vi "Make DLL Param(Read Batch Profile Rsp).vi"(1 "Read Batch Profile Rsp":T1) -> (0 "pRsp":T2)   [LabVIEW 2015, in "KEYENCE LJ-X8000A.lvlib"]
uses:
  KEYENCE LJ-X8000A.lvlib
  Public/Clusters/Read Batch Profile Rsp.ctl
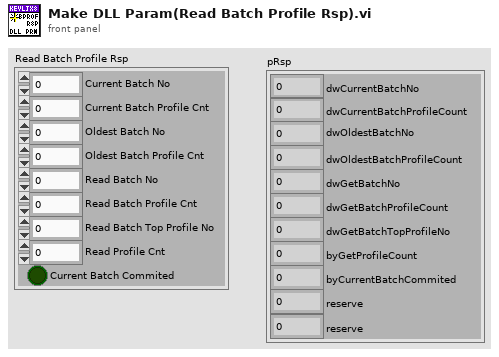
[diagram p1: front panel]
types:
  T1 = typedef "KEYENCE LJ-X8000A.lvlib/Read Batch Profile Rsp.ctl" = cluster{"Current Batch No":u32, "Current Batch Profile Cnt":u32, "Oldest Batch No":u32, "Oldest Batch Profile Cnt":u32, "Read Batch No":u32, "Read Batch Profile Cnt":u32, "Read Batch Top Profile No":u32, "Read Profile Cnt":u32, "Current Batch Commited":bool}
  T2 = cluster{"dwCurrentBatchNo":u32, "dwCurrentBatchProfileCount":u32, "dwOldestBatchNo":u32, "dwOldestBatchProfileCount":u32, "dwGetBatchNo":u32, "dwGetBatchProfileCount":u32, "dwGetBatchTopProfileNo":u32, "byGetProfileCount":u8, "byCurrentBatchCommited":u8, "reserve":u8, "reserve":u8}
  T3 = cluster{"Current Batch No":u32, "Current Batch Profile Cnt":u32, "Oldest Batch No":u32, "Oldest Batch Profile Cnt":u32, "Read Batch No":u32, "Read Batch Profile Cnt":u32, "Read Batch Top Profile No":u32, "Read Profile Cnt":u32, u8, "reserve":u8, "reserve":u8}
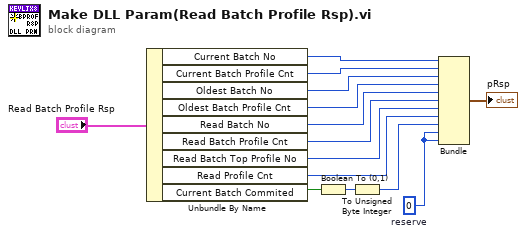
[diagram p0: block diagram]
diagram:
  w5 = u8 0  # reserve
  n1 = Unbundle By Name("Read Batch Profile Rsp") -> ("Current Batch No"=w14:u32, "Current Batch Profile Cnt"=w13:u32, "Oldest Batch No"=w12:u32, "Oldest Batch Profile Cnt"=w11:u32, "Read Batch No"=w10:u32, "Read Batch Profile Cnt"=w9:u32, "Read Batch Top Profile No"=w4:u32, "Read Profile Cnt"=w3:u32, "Current Batch Commited"=w7:bool)
  n2 = Boolean To (0,1)(Boolean=w7) -> (0, 1=w8:i16)
  n3 = To Unsigned Byte Integer(number=w8) -> (unsigned 8bit integer=w6:u8)
  n4 = Bundle("Current Batch No"=w14, "Current Batch Profile Cnt"=w13, "Oldest Batch No"=w12, "Oldest Batch Profile Cnt"=w11, "Read Batch No"=w10, "Read Batch Profile Cnt"=w9, "Read Batch Top Profile No"=w4, "Read Profile Cnt"=w3, w6, "reserve"=w5, "reserve"=w5) -> (→"pRsp":T3)  [unwired: 1 in]
